vi "run sequences.vi"(8 "error in (no error)":errorcluster, 9 "continue location":i32=-1, 10 "sequences":string[](array[string]), 11 "Simple Sequencer API in":refnum<class "Simple Sequencer API.lvclass">) -> (0 "error out":errorcluster, 3 "Simple Sequencer API out":refnum<class "Simple Sequencer API.lvclass">)   [LabVIEW 2014, in "Simple Sequencer API.lvclass"]
doc: "Runs one or more sequences specified by their sequence name. \n\nOnce all sequences in the array have completed, the 'continue location' specifies which sequence to continue executing (or loop) from. The default value of -1 indicates that the sequencer should stop after the last sequence completes."
uses:
  Simple Sequencer API.lvclass
  Simple Sequencer API.lvclass/Simple Sequencer API.ctl
  module/execution/meta sequence definition.ctl
  module/execution/sequencer commands.ctl
  <vilib>/NI/AMC/Create Single Message.vi
  <vilib>/NI/AMC/Update Message Routing Info.vi
  <vilib>/NI/AMC/Send Message.vi
  module/configuration/Simple Sequencer TBM configuration.lvclass
  module/execution/Simple Sequencer TBM runtime.lvclass
  <vilib>/NI/AMC/AMC.lvlib
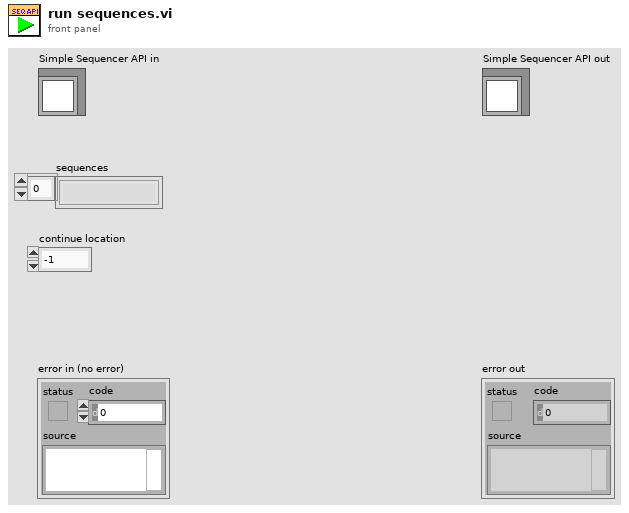
[diagram p1: front panel]
types:
  T1 = typedef "Simple Sequencer TBM runtime.lvclass/sequencer commands.ctl" = enum16{"Run", "Pause", "Resume", "Stop"}
  T2 = typedef "Simple Sequencer TBM runtime.lvclass/meta sequence definition.ctl" = cluster{"sequence length":i32, "sequence pointers":i32[], "continue location":i32}
  T3 = typedef "AMC.lvlib/Message Queue.ctl" = refnum<queue>
  T4 = typedef "Simple Sequencer TBM configuration.lvclass/sequence definition.ctl" = cluster{"sequence name":string, "action configs":refnum<class "action configuration.lvclass">[]}
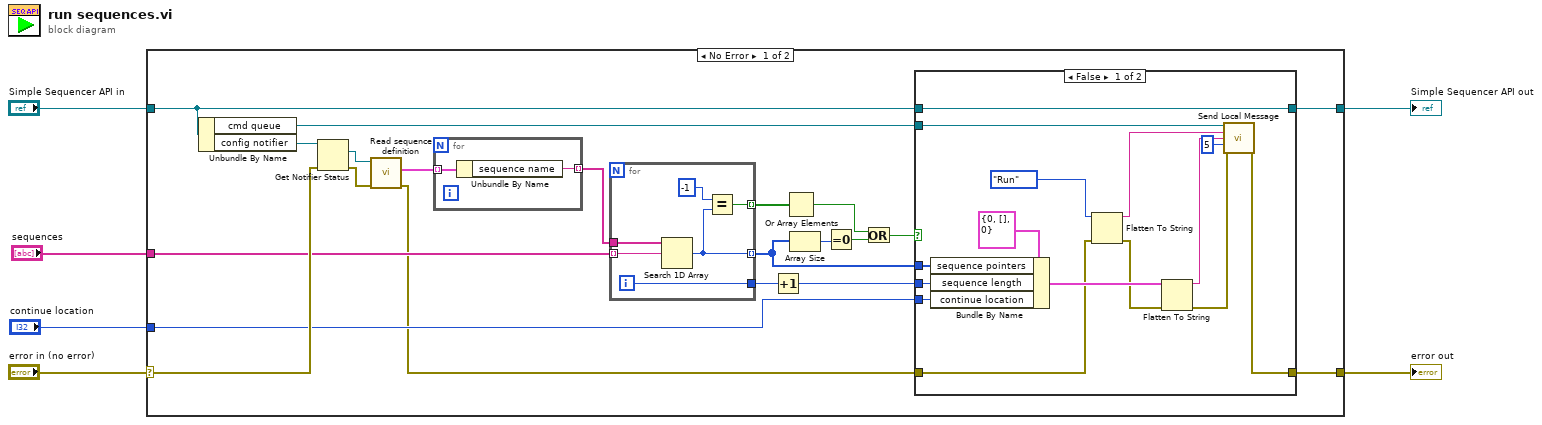
[diagram p0: block diagram]
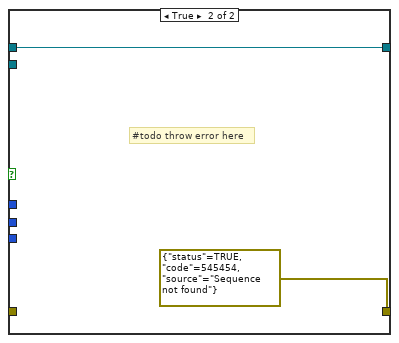
[diagram p2: hidden frame]
diagram:
  n1 = case shown="No Error" "error in (no error)" {
    selector: "error in (no error)" -> [w23 w54]
    tunnel: [w15 w54] -> w5
    tunnel: [w8 w53] -> w3
    tunnel: "Simple Sequencer API in" -> [w7 w53]
    tunnel: "sequences" -> [w21 _]
    tunnel: "continue location" -> [w18 _]
    frame No Error {
      n2 = Unbundle By Name(w7) -> ("cmd queue"=w17:T3, "config notifier"=w27:refnum<notifier>)
      n3 = Get Notifier Status(notifier=w27, error in (no error)=w23) -> (current notification=w26:refnum<class "Simple Sequencer TBM configuration.lvclass">, error out=w24:errorcluster)  [unwired: 3 out]
      n4 = call-dynamic "Read sequence definition.vi"("error in (no error)"=w24, "Simple Sequencer TBM configuration in"=w26) -> ("error out"=w16:errorcluster, "sequence definitions"=w25:T4[])  [unwired: 7 in, 1 out]
      n5 = for {
        tunnel: w25 -> [w52] mode=indexing
        tunnel: [w51] -> w22 mode=indexing
        n6 = Unbundle By Name(w52) -> ("sequence name"=w51:string)
      }
      n7 = for {
        tunnel: w22 -> [w50]
        tunnel: w21 -> [w49] mode=indexing
        tunnel: [w47] -> w13 mode=indexing
        tunnel: [w48] -> w20
        tunnel: [w45] -> w14 mode=indexing
        i -> [w48]
        n8 = Search 1D Array(1D array=w50, element=w49) -> (index of element=w47:i32)  [unwired: 1 in]
        n9 = Equal?(x=-1, y=w47) -> (x = y?=w45:bool)
      }
      n10 = Increment(x=w20) -> (x+1=w19:i32)
      n11 = Or Array Elements(Boolean array=w14) -> (logical OR=w10:bool)
      n12 = Array Size(array=w13) -> (size(s)=w12:i32)
      n13 = Equal To 0?(x=w12) -> (x = 0?=w11:bool)
      n14 = Or(x=w10, y=w11) -> (x .or. y?=w9:bool)
      n15 = case shown="False" w9 {
        tunnel: w19 -> [w41 _]
        tunnel: w18 -> [w40 _]
        tunnel: w17 -> [w39 _]
        tunnel: w16 -> [w31 _]
        tunnel: [w30 errorcluster {"status"=TRUE, "code"=545454, "source"="Sequence not found"} ("error out")] -> w15
        tunnel: w13 -> [w29 _]
        tunnel: [w28 w44] -> w8
        tunnel: w7 -> [w28 w44]
        frame False {
          n16 = Bundle By Name(cluster=T2 {"sequence length"=0, "sequence pointers"=[], "continue location"=0} ("meta sequence definition"), "sequence pointers"=w29, "sequence length"=w41, "continue location"=w40) -> (w37:T2)
          n17 = Flatten To String(anything=sequencer_commands."Run" ("Commands"), error in (no error)=w31) -> (data string=w34:string, error out=w36:errorcluster)  [unwired: 2 in, 1 out]
          n18 = Flatten To String(anything=w37, error in (no error)=w36) -> (data string=w33:string, error out=w35:errorcluster)  [unwired: 2 in, 1 out]
          n19 = call <vilib>:"Send Local Message.vi"("message queue in"=w39, "message name"=w34, "message value"=w33, "timeout (-1 ms)"=5, "error in"=w35) -> ("error out"=w30:errorcluster)  [unwired: 8 in, 2 out]
        }
        frame True {
          # "#todo throw error here"
        }
      }
    }
    frame Error {
    }
  }
  "error out" <- w5
  "Simple Sequencer API out" <- w3
